vi "Read Status.vi"(8 "error in (no error)":errorcluster, 11 "HttpDownloadTask in":T2) -> (0 "error out":errorcluster, 1 "Progress":dbl, 2 "RunningStats":T1, 3 "HttpDownloadTask out":T2, 4 "Done or Error":bool)   [LabVIEW 2018, in "LabVIEWHTTPClient_NET.lvlib" / "HttpDownloadTask.lvclass"]
uses:
  HttpDownloadTask.lvclass
  Types/DownloadTask_ref.ctl
  Types/DownloadStats_Cluster.ctl
  HttpDownloadTask.lvclass/HttpDownloadTask.ctl
  Types/HttpNet_error_enum.ctl
  HttpContent/HttpContent.lvclass
  LabVIEWHTTPClient_NET.lvlib
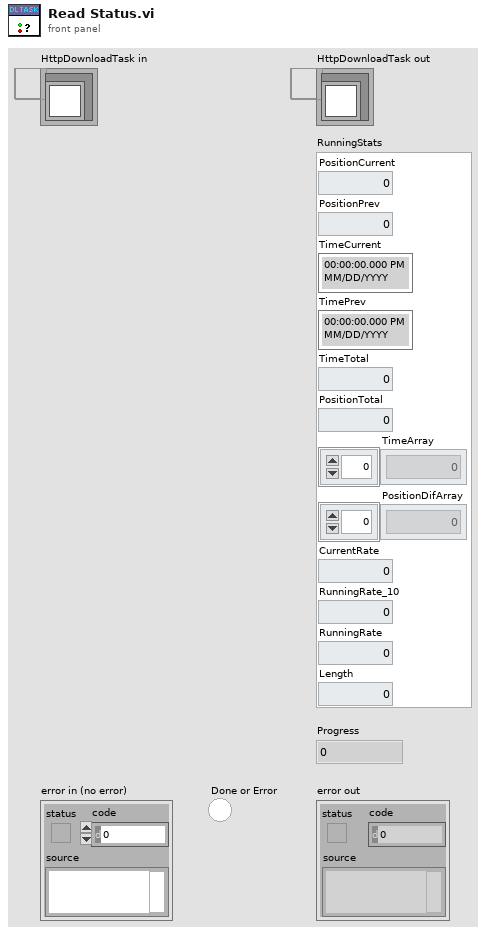
[diagram p1: front panel]
types:
  T1 = typedef "LabVIEWHTTPClient_NET.lvlib/DownloadStats_Cluster.ctl" = cluster{"PositionCurrent":dbl, "PositionPrev":dbl, "TimeCurrent":timestamp, "TimePrev":timestamp, "TimeTotal":dbl, "PositionTotal":dbl, "TimeArray":dbl[], "PositionDifArray":dbl[], "CurrentRate":dbl, "RunningRate_10":dbl, "RunningRate":dbl, "Length":dbl}
  T2 = typedef "LabVIEWHTTPClient_NET.lvlib/HttpDownloadTask.lvclass/DownloadTask_ref.ctl" = refnum<data-value>
  T3 = typedef "LabVIEWHTTPClient_NET.lvlib/HttpNet_error_enum.ctl" = enum16{"REST method is not available", "URL cannot be blank", "Output filepath cannot be empty", "Input filepath cannot be empty", "Internal .NET error %s", "Output filepath cannot be directory", "Download Task no longer exists", "Mutipart Put not supported from REST Client Interface.  Please revert to lower level classes"}
  T4 = typedef "LabVIEWHTTPClient_NET.lvlib/ScaledValue_ring.ctl" = u64
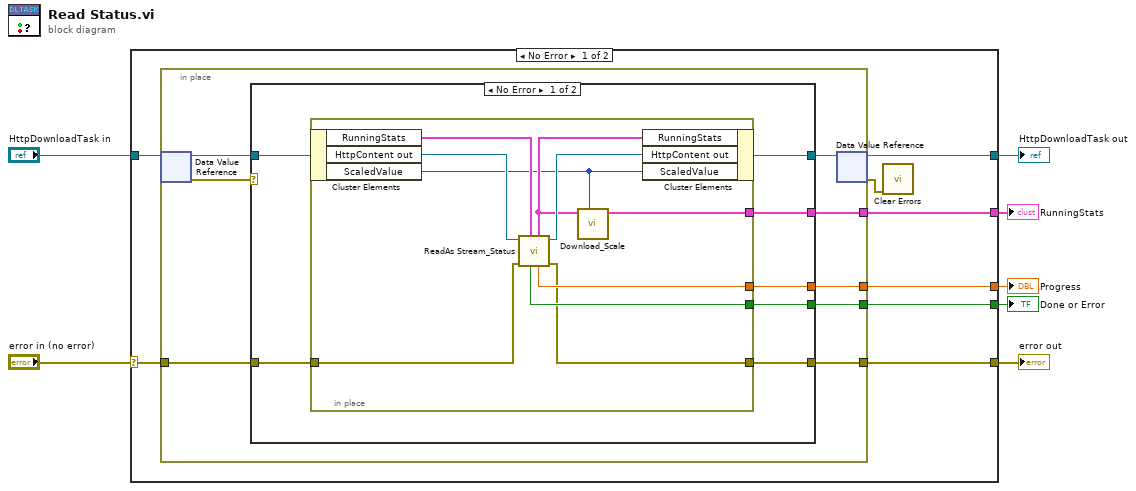
[diagram p0: block diagram]
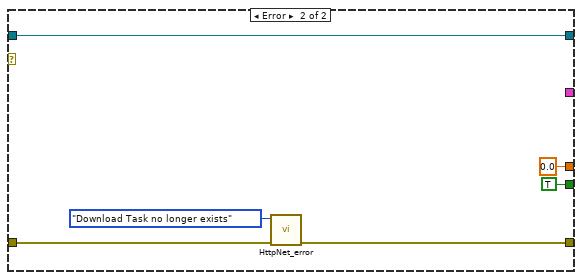
[diagram p2: hidden frame]
diagram:
  n1 = case shown="No Error" "error in (no error)" {
    selector: "error in (no error)" -> [w12 w48]
    tunnel: [w11 w48] -> w6
    tunnel: [w9 w47] -> w4
    tunnel: "HttpDownloadTask in" -> [w10 w47]
    tunnel: [w15 _] -> w3
    tunnel: [w14 _] -> w2
    tunnel: [w13 _] -> w1
    frame No Error {
      n2 = in-place {
        in-place-border: [w23] -> w15
        in-place-border: [w22] -> w14
        in-place-border: [w21] -> w13
        in-place-border: w12 -> [w20]
        in-place-border: [w19] -> w11
        n3 = in-place-dvr #1(w10) -> (w18:refnum<class "HttpDownloadTask.lvclass">, w16:errorcluster)
        n4 = case shown="No Error" w16 {
          tunnel: [w30 _] -> w23
          tunnel: [w29 0.0 ("Progress")] -> w22
          tunnel: [w28 TRUE ("Done or Error")] -> w21
          tunnel: w20 -> [w27 w43]
          tunnel: [w26 w42] -> w19
          tunnel: w18 -> [w25 w44]
          tunnel: [w24 w44] -> w17
          frame No Error {
            n5 = in-place {
              in-place-border: [w35] -> w30
              in-place-border: [w34] -> w29
              in-place-border: [w33] -> w28
              in-place-border: w27 -> [w32]
              in-place-border: [w31] -> w26
              n6 = in-place-cluster #2(w25) -> ("RunningStats"=w38:T1, "HttpContent out"=w40:refnum<class "HttpContent.lvclass">, "ScaledValue"=w36:T4)
              n7 = call "ReadAs Stream_Status.vi"("DownloadStats In"=w38, "error in (no error)"=w32, "HttpContent in"=w40) -> ("error out"=w31:errorcluster, "HttpContent out"=w39:refnum<class "HttpContent.lvclass">, "Progress"=w34:dbl, "RunningStats Out"=w37:T1, "Done or Error"=w33:bool)  [unwired: 2 in, 2 out]
              n8 = call "Download_Scale.vi"("ScaledValue"=w36, "DownloadStats In"=w37) -> ("RunningStats"=w35:T1)  [unwired: 9 in]
              n9 = in-place-cluster #2("RunningStats"=w37, "HttpContent out"=w39, "ScaledValue"=w36) -> (w24:refnum<class "HttpDownloadTask.lvclass">)
            }
          }
          frame Error {
            n10 = call "HttpNet_error.vi"("Error In"=w43, "Error"=HttpNet_error_enum."Download Task no longer exists") -> ("Error Out"=w42:errorcluster)  [unwired: 9 in]
          }
        }
        n11 = in-place-dvr #1(w17) -> (w9:T2, w8:errorcluster)
      }
      n12 = call <vilib>:"Clear Errors.vi"("error in (no error)"=w8) -> ()  [unwired: 5 in, 2 out]
    }
    frame Error {
    }
  }
  "error out" <- w6
  "HttpDownloadTask out" <- w4
  "RunningStats" <- w3
  "Progress" <- w2
  "Done or Error" <- w1
